vi "init.vi"(8 "error in (no error)":errorcluster, 9 "Size":u32, 10 "Array":T1[](array[typedef]), 11 "Bucket in":refnum<class "Bucket.lvclass">) -> (0 "error out":errorcluster, 3 "Bucket out":refnum<class "Bucket.lvclass">)   [LabVIEW 2017, in "Bucket.lvclass"]
uses:
  <userlib>/836-Library/Data_Structures/HashMap/Support/Bucket/Bucket.lvclass
  <userlib>/836-Library/Data_Structures/HashMap/Support/Bucket/Types/KeyValuePair.ctl
  <userlib>/836-Library/Data_Structures/HashMap/Support/Bucket/Bucket.lvclass/Bucket.ctl
  <vilib>/Utility/error.llb/Error Cluster From Error Code.vi
  <vilib>/ErrorRing/Error Ring.xnode
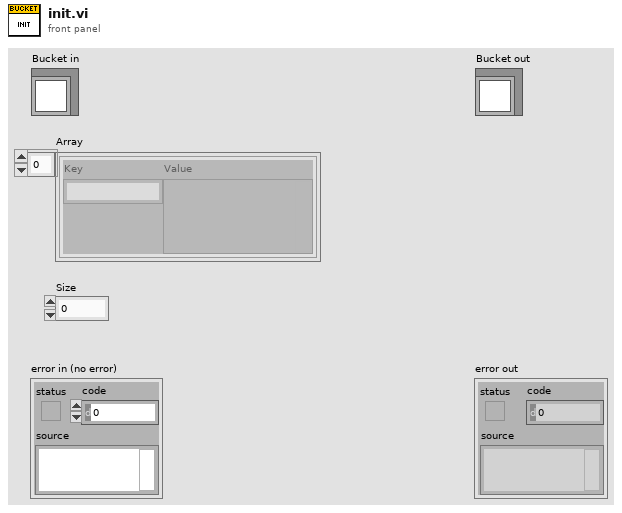
[diagram p1: front panel]
types:
  T1 = typedef "KeyValuePair.ctl" = cluster{"Key":string, "Value":variant}
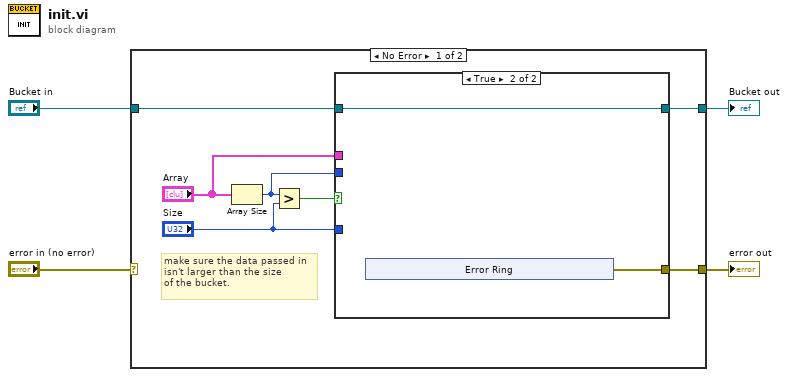
[diagram p0: block diagram]
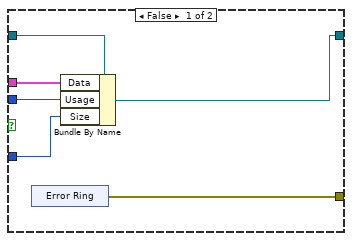
[diagram p2: hidden frame]
diagram:
  n1 = case shown="No Error" "error in (no error)" {
    selector: "error in (no error)" -> [_ w27]
    tunnel: [w8 w27] -> w3
    tunnel: [w9 w26] -> w1
    tunnel: "Bucket in" -> [w10 w26]
    frame No Error {
      # "make sure the data passed in\nisn't larger than the size\nof the bucket."
      n2 = Array Size(array="Array") -> (size(s)=w5:i32)
      n3 = Greater?(x=w5, y="Size") -> (0:w11:bool)
      n4 = case shown="True" w11 {
        tunnel: w10 -> [w17 w20]
        tunnel: [w12 w20] -> w9
        tunnel: [w13 w19] -> w8
        tunnel: "Array" -> [w16 _]
        tunnel: "Size" -> [w15 _]
        tunnel: w5 -> [w14 _]
        frame False {
          n5 = xnode "Error Ring"() -> ("error out"=w13:errorcluster)
          n6 = Bundle By Name(cluster=w17, "Data"=w16, "Usage"=w14, "Size"=w15) -> (w12:refnum<class "Bucket.lvclass">)
        }
        frame True {
          n7 = xnode "Error Ring"() -> ("error out"=w19:errorcluster)
        }
      }
    }
    frame Error {
    }
  }
  "error out" <- w3
  "Bucket out" <- w1
